vi "Autonomous Independent (1).vi"() -> ()   [LabVIEW 2016]
doc: "This VI is called when autonomous begins, and will automatically be terminated when autonomous ends. You can carry out timed or sensor driven robot movement independently without needing to return to the caller."
uses:
  <vilib>/Rock Robotics/WPI/Utilities/WPI_GetSetVariantRefNum.vi
  <vilib>/Rock Robotics/Network Tables/NT Read String.vi
  <vilib>/Rock Robotics/Network Tables/NT Write Numeric Array.vi
  <vilib>/Rock Robotics/WPI/RobotDrive/WPI_RobotDriveArcadeDrive_Standard(NoSaturation).vi
  Robot Global Data.vi
  <vilib>/Rock Robotics/Network Tables/NT Write Number.vi
  <vilib>/Rock Robotics/WPI/Counter/WPI_CounterDigitalInputToDigitalSource.vi
  <vilib>/Rock Robotics/SystemInterfaces/DIO/FPGA_DIOChannel.ctl
panel:
  out "Hook found 2":bool
  out "Degrees to turn 2":dbl
  out "Pixels to turn 2":dbl
  out "Hook Center 2":dbl
  out "Initial Hook Center 3":dbl
  out "Initial Hook Found 2":bool
  out "Distance to wall (in) 2":dbl
  out "Hook Center Cons":dbl
  out "Initial Hook Center 2":dbl
  out "Hook Center":dbl
  out "Initial Hook Found":bool
  out "Pixels to turn":dbl
  out "Move forward? S 5":bool
  out "Move forward? S4":bool
  out "Move forward? S 3":bool
  out "Move forward? S2":bool
  out "Move forward? S1":bool
  out "Distance to wall (in)":dbl
  out "Degrees to turn":dbl
  out "Hook found":bool
  out "gyro":dbl
  out "sonar distance (inches)":dbl
  out "Hook Found In False Case 2":bool
  out "gyro step  four":dbl
  out "gyro step  three":dbl
  out "gyro step two":dbl
  out "gyro step one":dbl
  out "Step 3":bool
  out "Step 2":bool
  out "Step 1":bool
  out "Encoder Loop":dbl
  out "Encoder Loop":string
  out "S2 Encoder":dbl
  out "Encoder Direction 2":string
  out "S1 Encoder inches":dbl
  out "Encoder Direction":string
  out "Current Movement, for debugging 2":T1 {"Y Joystick Value" scale=1.0..-1.0; "X Joystick Value" scale=-1.0..1.0}
  in  "Array of robot movements 2":T2(array[cluster])=[{"X Joystick Value"=0.39393939393939403, "Y Joystick Value"=0.0, "Delay (sec)"=1.0, "Movement Name"="turn"}, {"X Joystick Value"=-0.3737373737373737, "Y Joystick Value"=0.0, "Delay (sec)"=1.0, "Movement Name"="turn back"}] {"Y Joystick Value" scale=1.0..-1.0; "X Joystick Value" scale=-1.0..1.0}
  out "Motor Values":dbl[](array[numeric])
  out "Switch Pressed":bool
  out "Current Movement, for debugging":T1 {"Y Joystick Value" scale=1.0..-1.0; "X Joystick Value" scale=-1.0..1.0}
  in  "Array of robot movements":T2(array[cluster])=[{"X Joystick Value"=0.39393939393939403, "Y Joystick Value"=0.0, "Delay (sec)"=1.0, "Movement Name"="turn"}, {"X Joystick Value"=-0.3737373737373737, "Y Joystick Value"=0.0, "Delay (sec)"=1.0, "Movement Name"="turn back"}] {"Y Joystick Value" scale=1.0..-1.0; "X Joystick Value" scale=-1.0..1.0}
  # "Sensor Readings\nConstanly updated in\nwhile loopes"
  # "Be sure to right-click and choose Data Operations>>Make Current Value default if you want to save the array values with the VI"
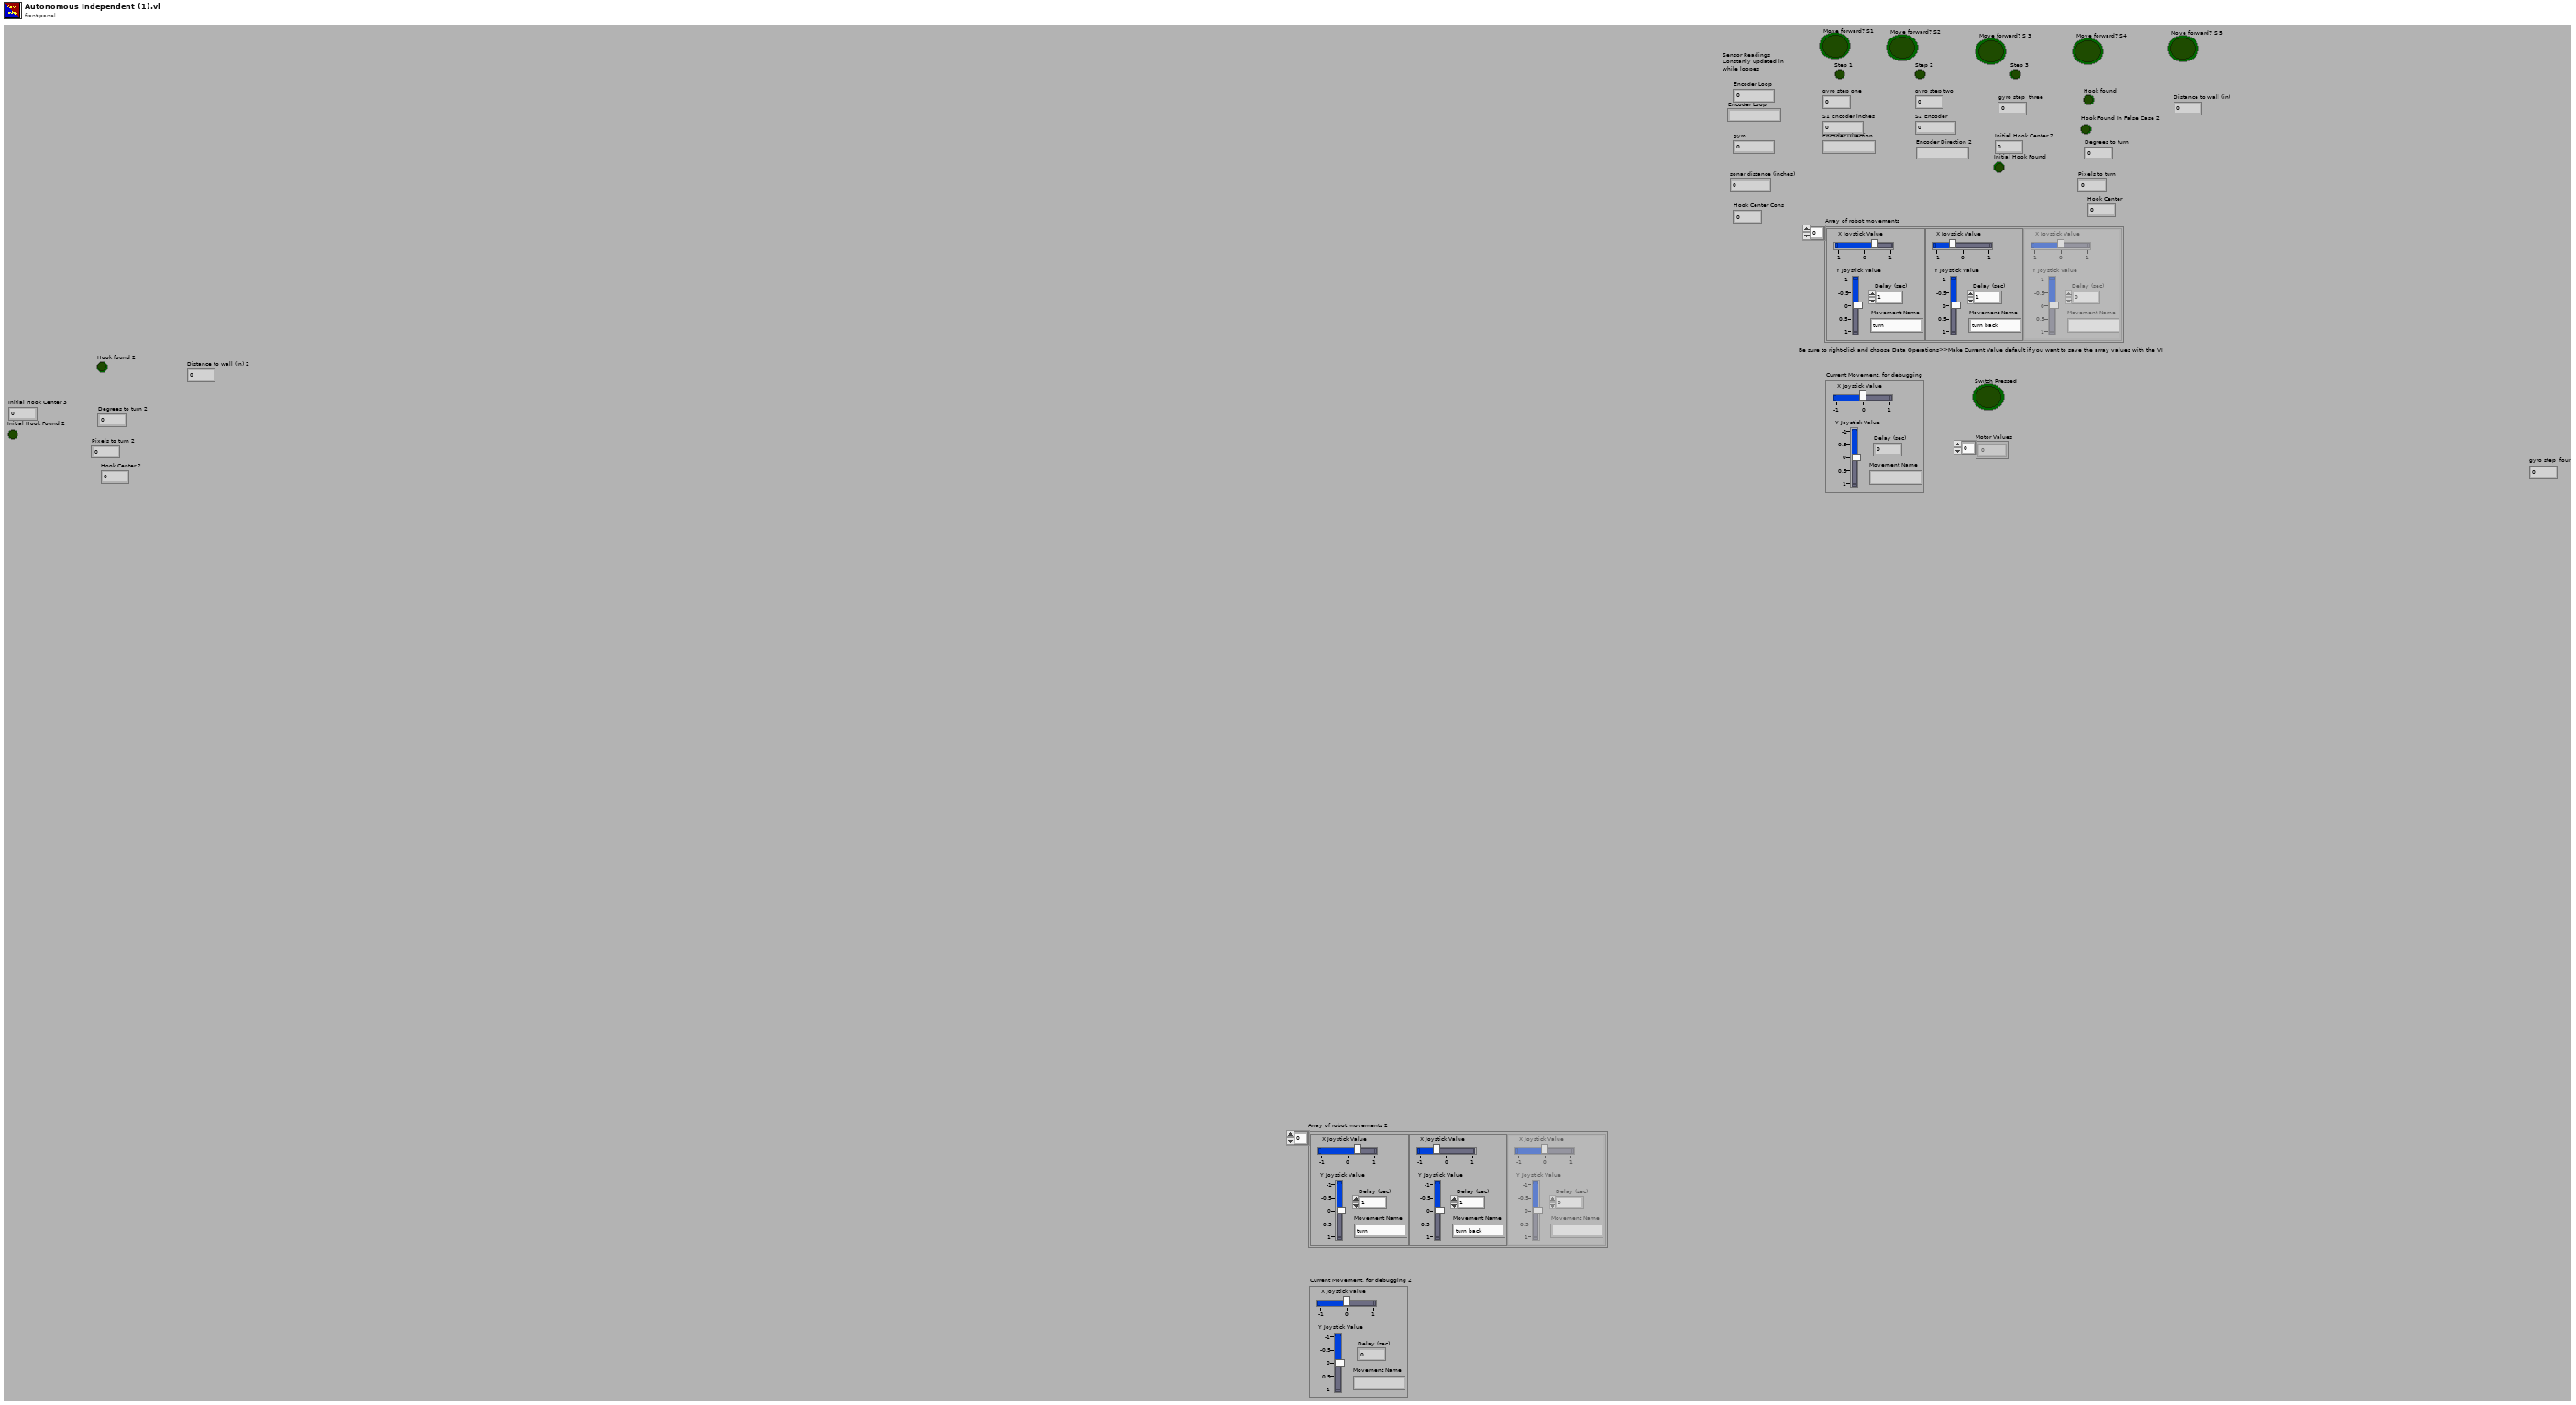
[diagram p1: front panel]
types:
  T1 = cluster{"X Joystick Value":dbl, "Y Joystick Value":dbl, "Delay (sec)":dbl, "Movement Name":string}
  T2 = cluster{"X Joystick Value":dbl, "Y Joystick Value":dbl, "Delay (sec)":dbl, "Movement Name":string}[]
  T3 = typedef "FPGA_DIOChannel.ctl" = enum8{"DIO 0", "DIO 1", "DIO 2", "DIO 3", "DIO 4", "DIO 5", "DIO 6", "DIO 7", "DIO 8", "DIO 9", "DIO MXP 0", "DIO MXP 1", "DIO MXP 2", "DIO MXP 3", "DIO MXP 4", "DIO MXP 5", "DIO MXP 6", "DIO MXP 7", "DIO MXP 8", "DIO MXP 9", "DIO MXP 10", "DIO MXP 11", "DIO MXP 12", "DIO MXP 13", "DIO MXP 14", "DIO MXP 15", "SPI Port CS1", "SPI Port CS2", "SPI Port CS3", "SPI Port MISO", "SPI Port MOSI", "Invalid"}
  T4 = typedef "WPI_DigitalInputDevRef.ctl" = cluster{"DevStatus":errorcluster, "DIO Channel":T3}
  T5 = typedef "FPGA_CounterEncoderSourceConvertionLVSourceType.ctl" = cluster{"DevStatus":errorcluster, "AnalogTriggerMode?":bool, "DigitalMode":cluster{"DIO Channel":T6}, "AnalogTriggerMode":cluster{"AnalogTriggerIndex":T7, "OutputType":T8}}
  T6 = typedef "FPGA_DIODigitalSourceChannel.ctl" = enum8{"DIO 0", "DIO 1", "DIO 2", "DIO 3", "DIO 4", "DIO 5", "DIO 6", "DIO 7", "DIO 8", "DIO 9", "DIO MXP 0", "DIO MXP 1", "DIO MXP 2", "DIO MXP 3", "DIO MXP 4", "DIO MXP 5", "DIO MXP 6", "DIO MXP 7", "DIO MXP 8", "DIO MXP 9", "DIO MXP 10", "DIO MXP 11", "DIO MXP 12", "DIO MXP 13", "DIO MXP 14", "DIO MXP 15", "Disabled"}
  T7 = typedef "FPGA_AnalogTriggerIndex.ctl" = enum8{"Trig 0", "Trig 1", "Trig 2", "Trig 3", "Trig 4", "Trig 5", "Trig 6", "Trig 7", "Invalid"}
  T8 = typedef "FPGA_AnalogTriggerOutType.ctl" = enum16{"InWindow", "TriggerState", "Rising", "Falling"}
  T9 = typedef "WPI_EncoderDevRef.ctl" = cluster{"DevStatus":errorcluster, "EncoderIndex":T10, "CounterIndex":T11, "DistancePerCount":dbl, "Decoding Type":T12}
  T10 = typedef "FPGA_EncoderIdx.ctl" = enum8{"Enc 0", "Enc 1", "Enc 2", "Enc 3", "Enc 4", "Enc 5", "Enc 6", "Enc 7", "Invalid"}
  T11 = typedef "FPGA_CounterCtrSystemIndex.ctl" = enum8{"Ctr 0", "Ctr 1", "Ctr 2", "Ctr 3", "Ctr 4", "Ctr 5", "Ctr 6", "Ctr 7", "Invalid"}
  T12 = typedef "WPI_EncoderType.ctl" = enum16{"1x", "2x", "4x"}
  T13 = typedef "WPI_JoystickDevRef.ctl" = cluster{"Device":T14}
  T14 = typedef "WPI_JoystickDeviceEnum.ctl" = enum16{"USB 0", "USB 1", "USB 2", "USB 3", "USB 4", "USB 5"}
  T15 = typedef "WPI_DriverStationPositionInfo.ctl" = enum16{"1", "2", "3"}
  T16 = typedef "WPI_RobotDriveDevRef.ctl" = cluster{"DevStatus":errorcluster, "Motors[]":T17[], "Square Inputs":bool, "Max Output":dbl}
  T17 = typedef "WPI_MotorControlDeviceRef.ctl" = cluster{"DeviceStatus":errorcluster, "Type":T18, "PWM":cluster{"PWM Channel":T19, "DeadBand":T20}, "CAN":cluster{"Device Number":u8, "SetOutput VI Ref":variant, "GetOutput VI Ref":variant, "Enable VI Ref":variant, "Disable VI Ref":variant, "Data":variant}, "Invert":bool}
  T18 = typedef "WPI_MotorControlType.ctl" = enum16{"PWM", "CAN"}
  T19 = typedef "FPGA_DIOPWMChannel.ctl" = enum8{"PWM 0", "PWM 1", "PWM 2", "PWM 3", "PWM 4", "PWM 5", "PWM 6", "PWM 7", "PWM 8", "PWM 9", "PWM MXP 0", "PWM MXP 1", "PWM MXP 2", "PWM MXP 3", "PWM MXP 4", "PWM MXP 5", "PWM MXP 6", "PWM MXP 7", "PWM MXP 8", "PWM MXP 9", "Invalid"}
  T20 = typedef "WPI_PWMDeadband.ctl" = cluster{"Name":string, "maxPositivePwm":i32, "minPositivePwm":i32, "centerPwm":i32, "maxNegativePwm":i32, "minNegativePwm":i32, "angularRange":u16}
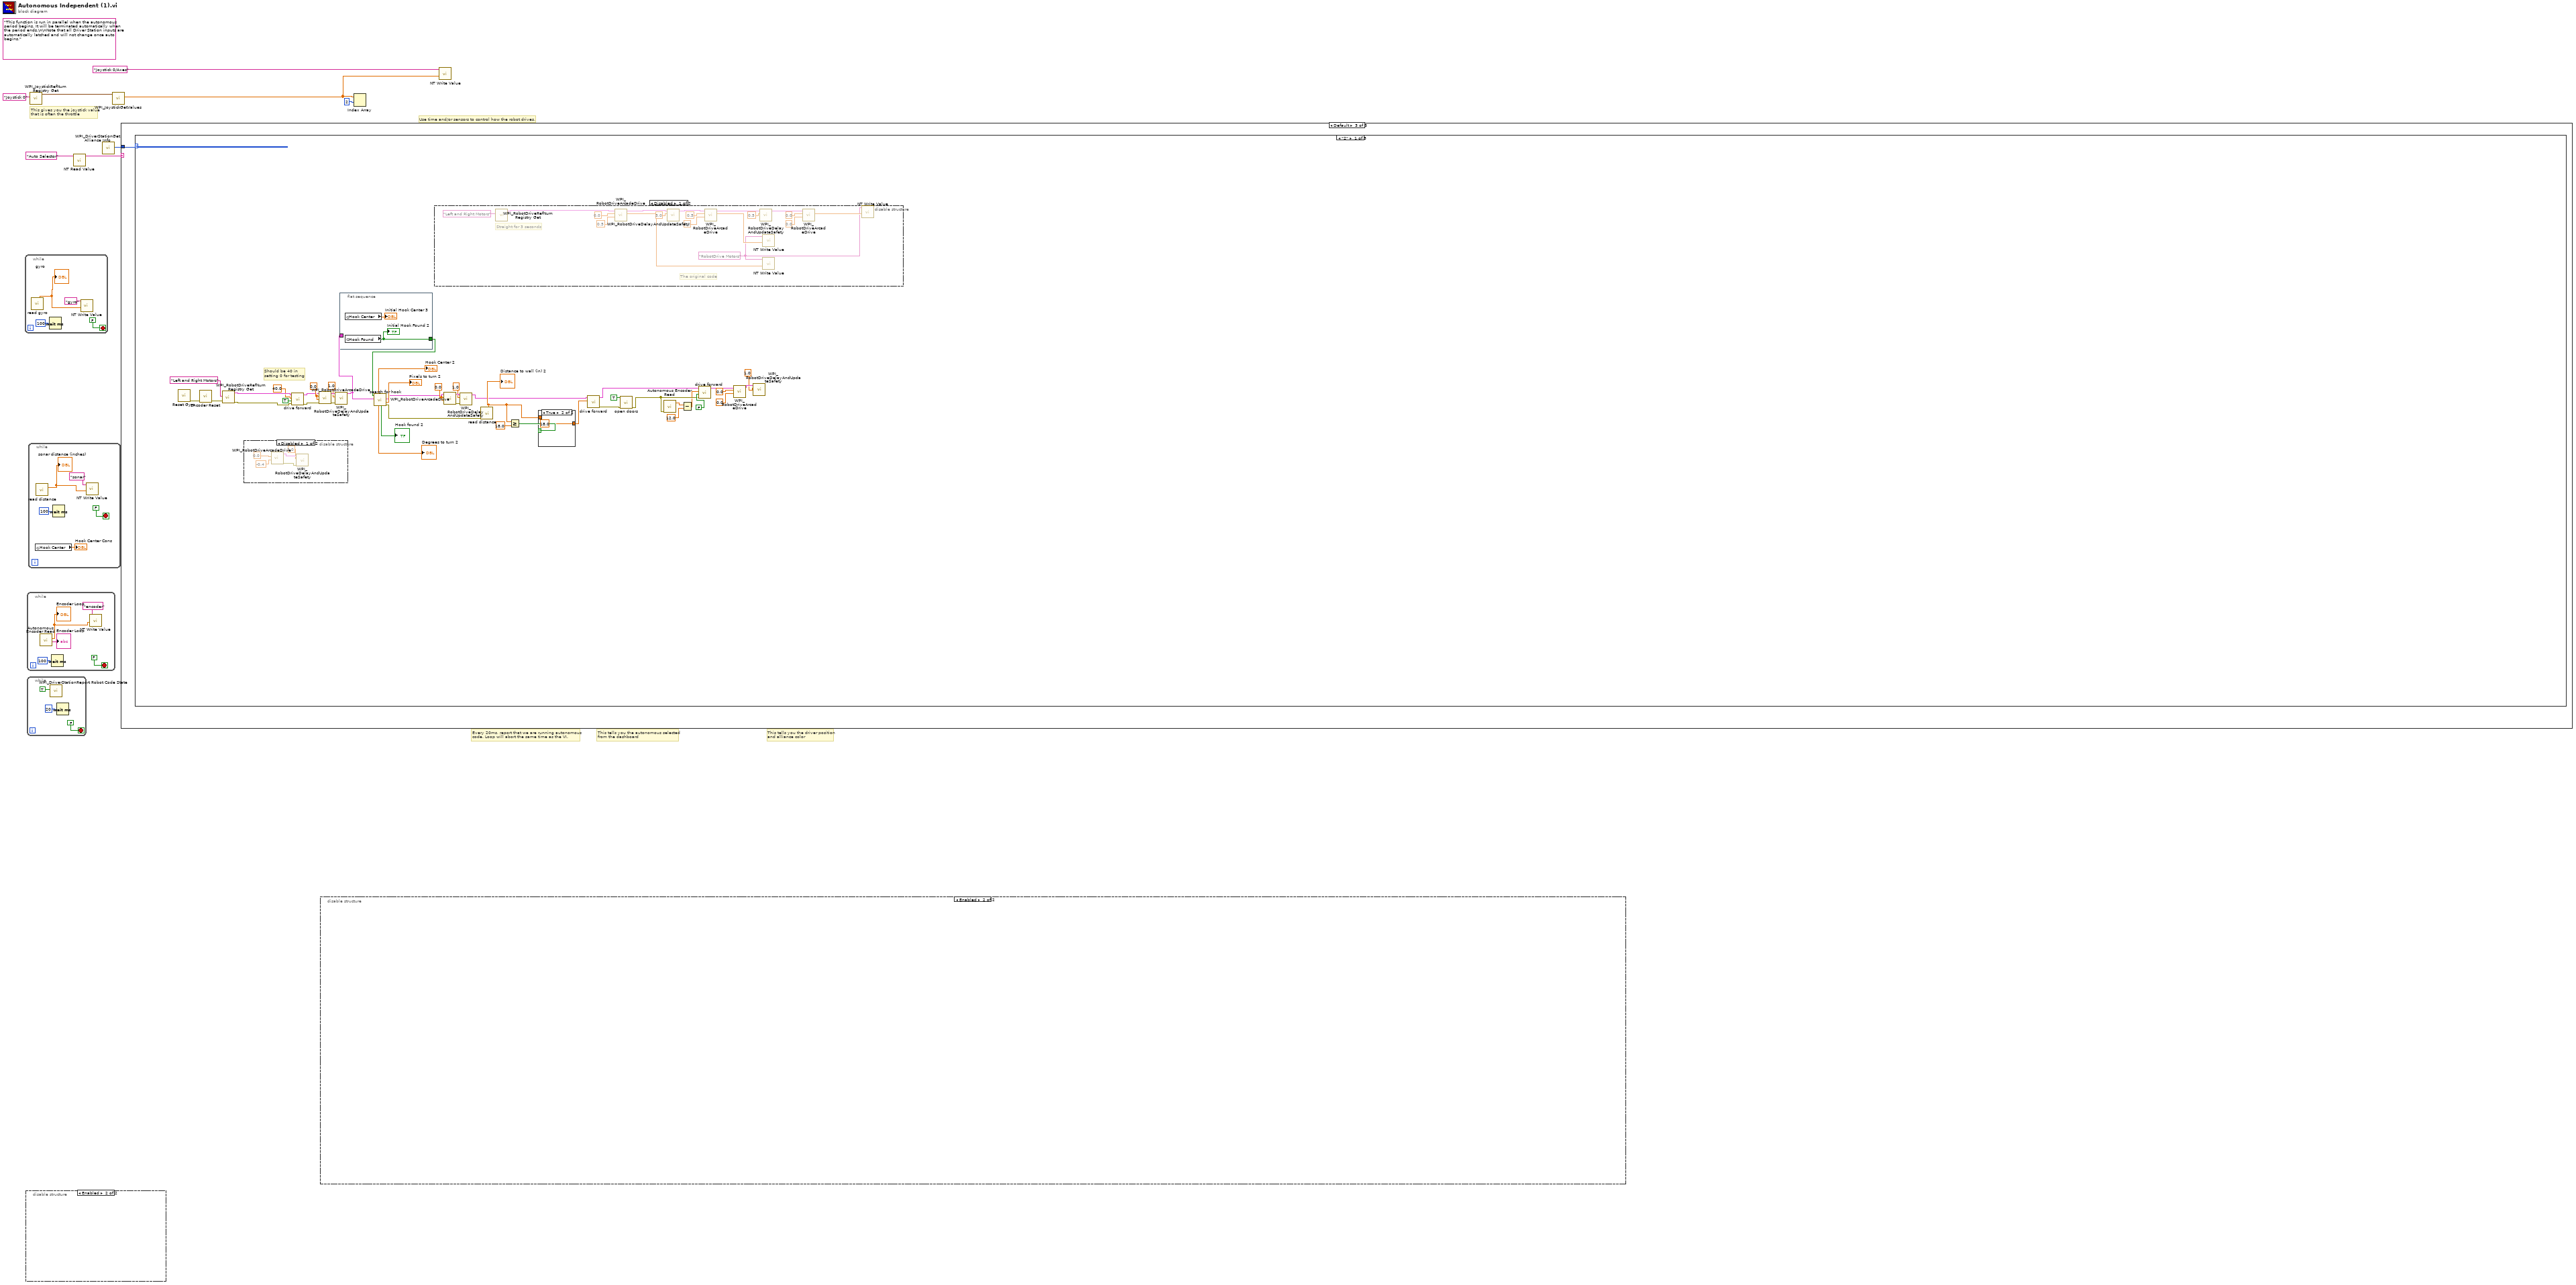
[diagram p0: block diagram]
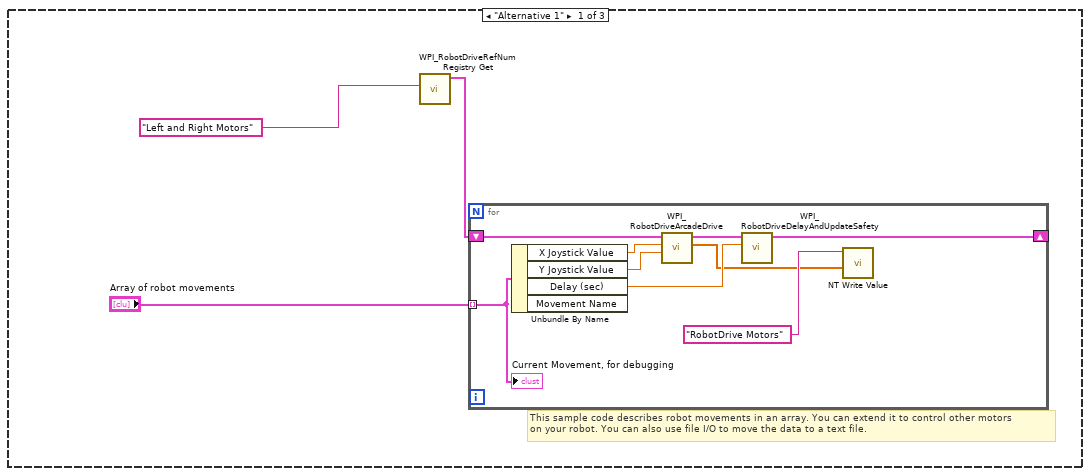
[diagram p2: hidden frame]
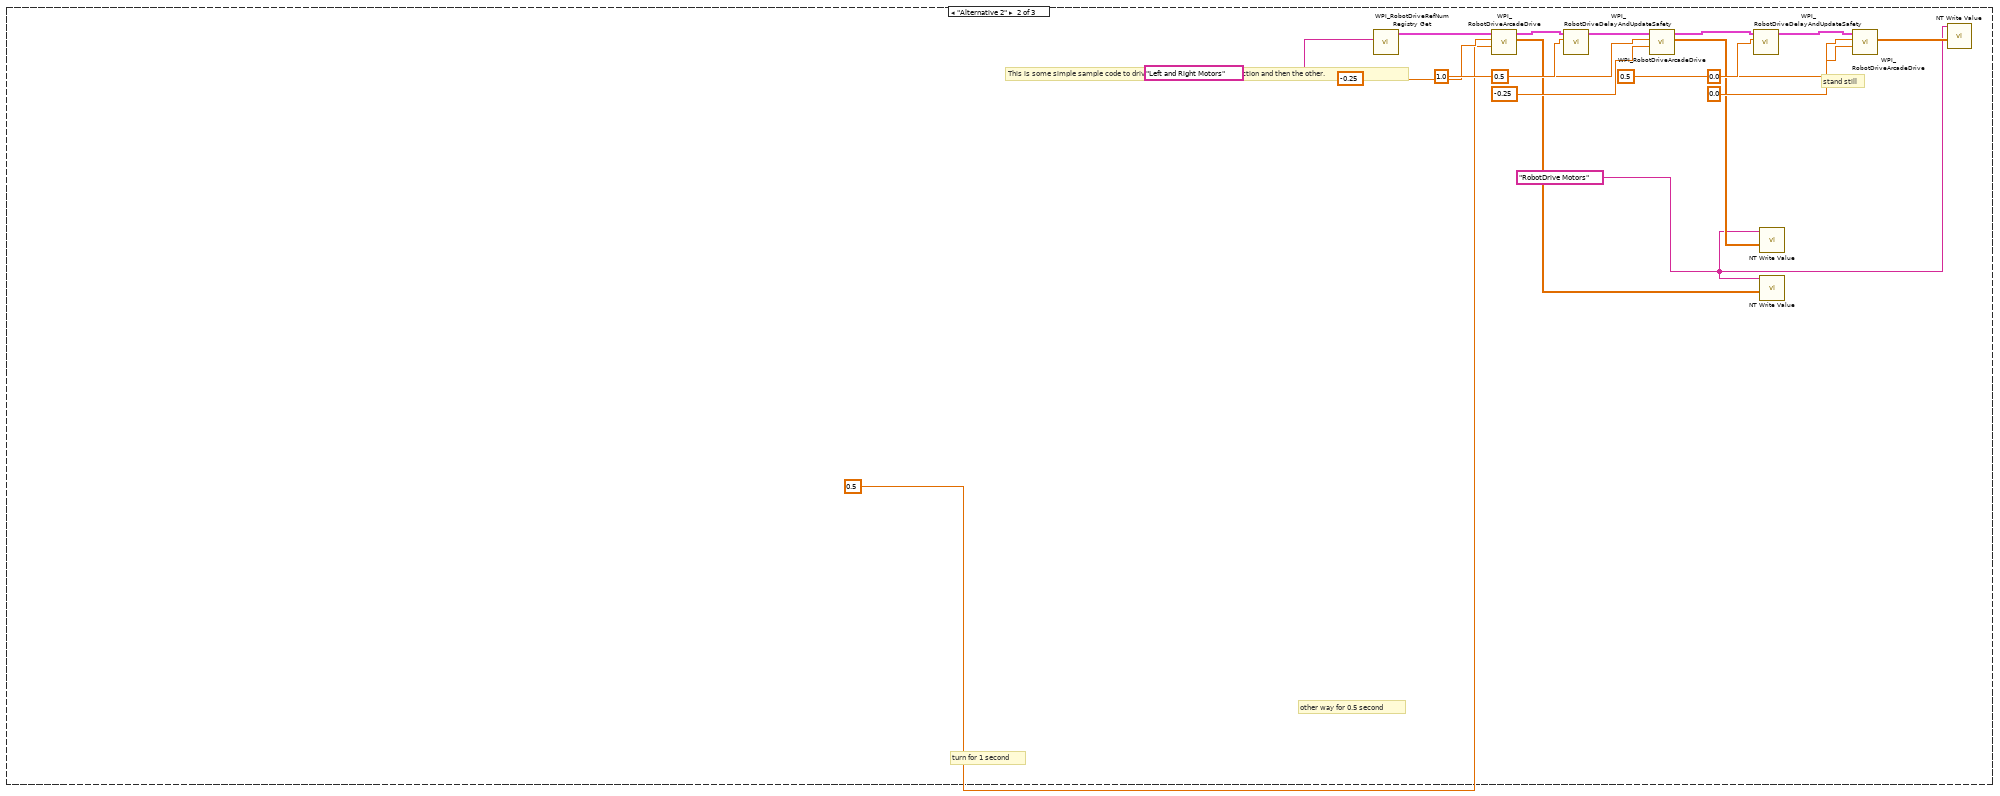
[diagram p3: hidden frame]
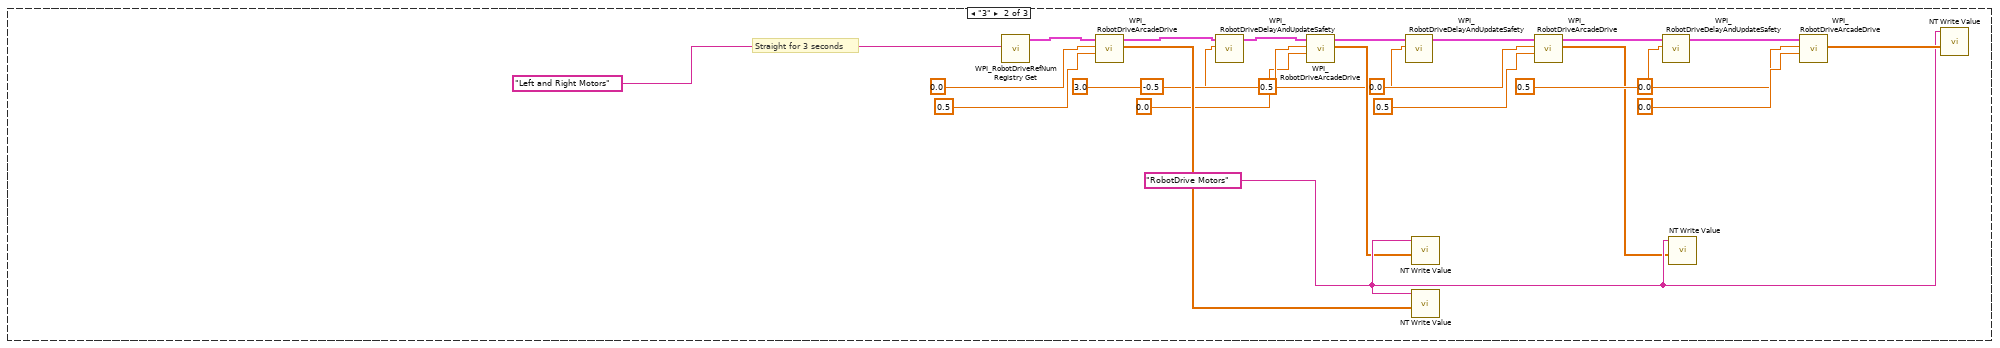
[diagram p7: hidden frame]
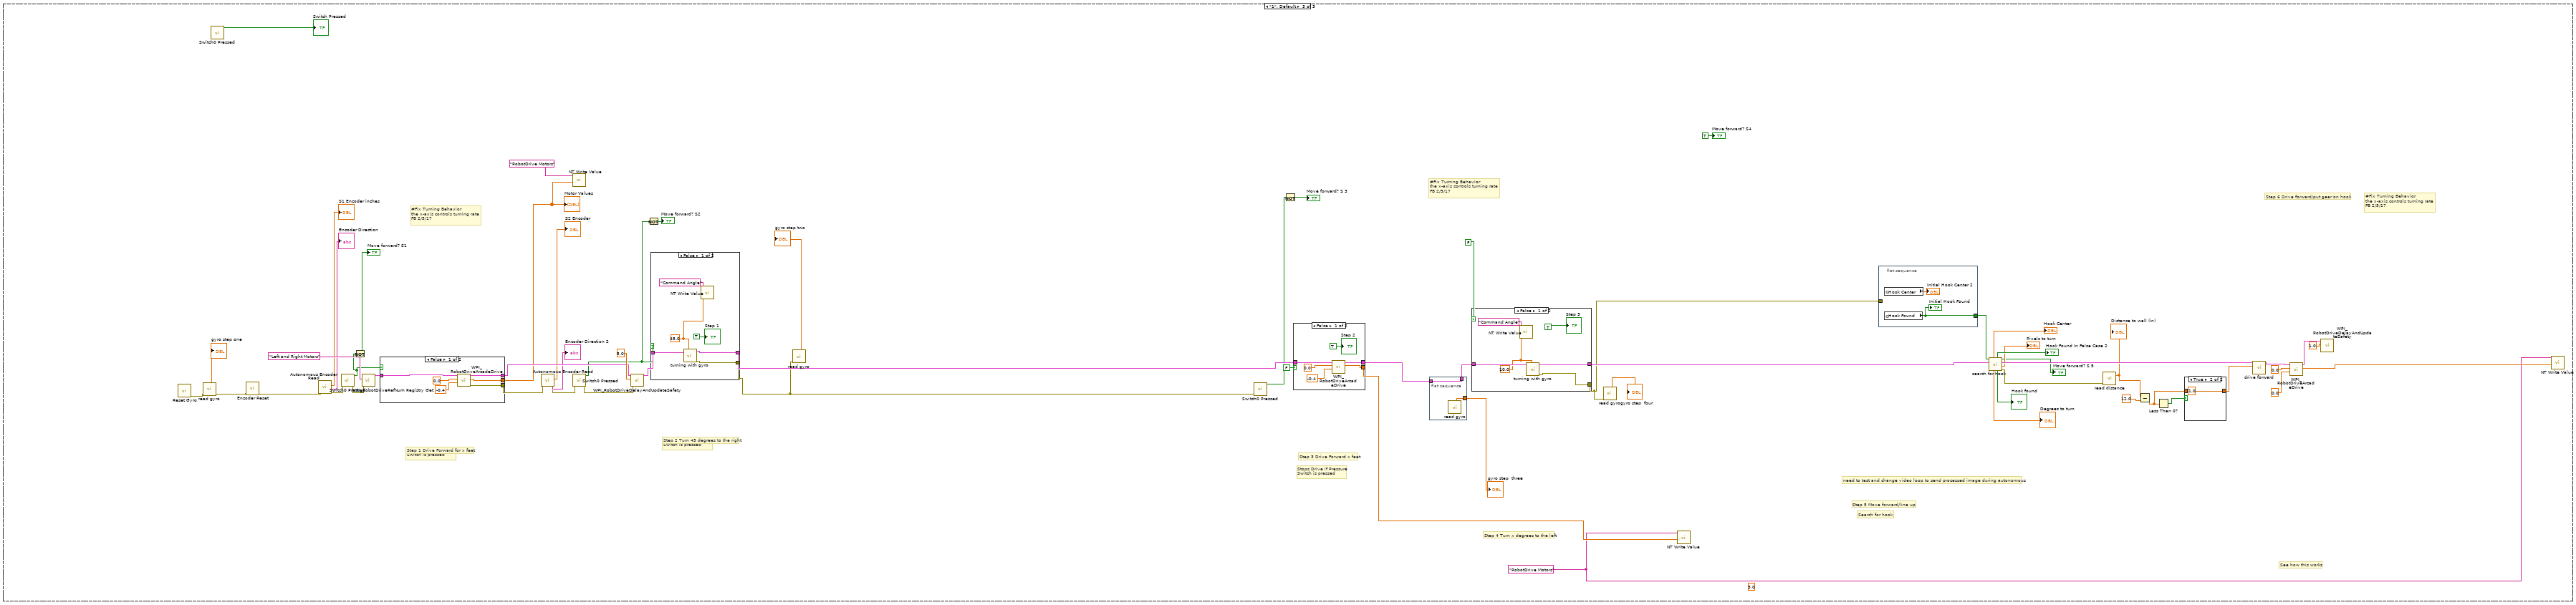
[diagram p8: hidden frame]
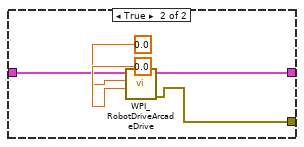
[diagram p10: hidden frame]
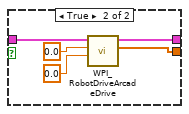
[diagram p11: hidden frame]
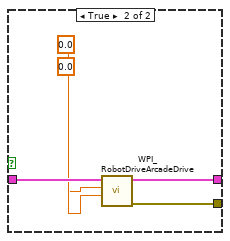
[diagram p12: hidden frame]
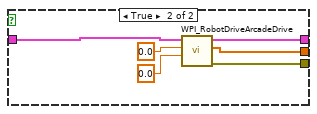
[diagram p13: hidden frame]
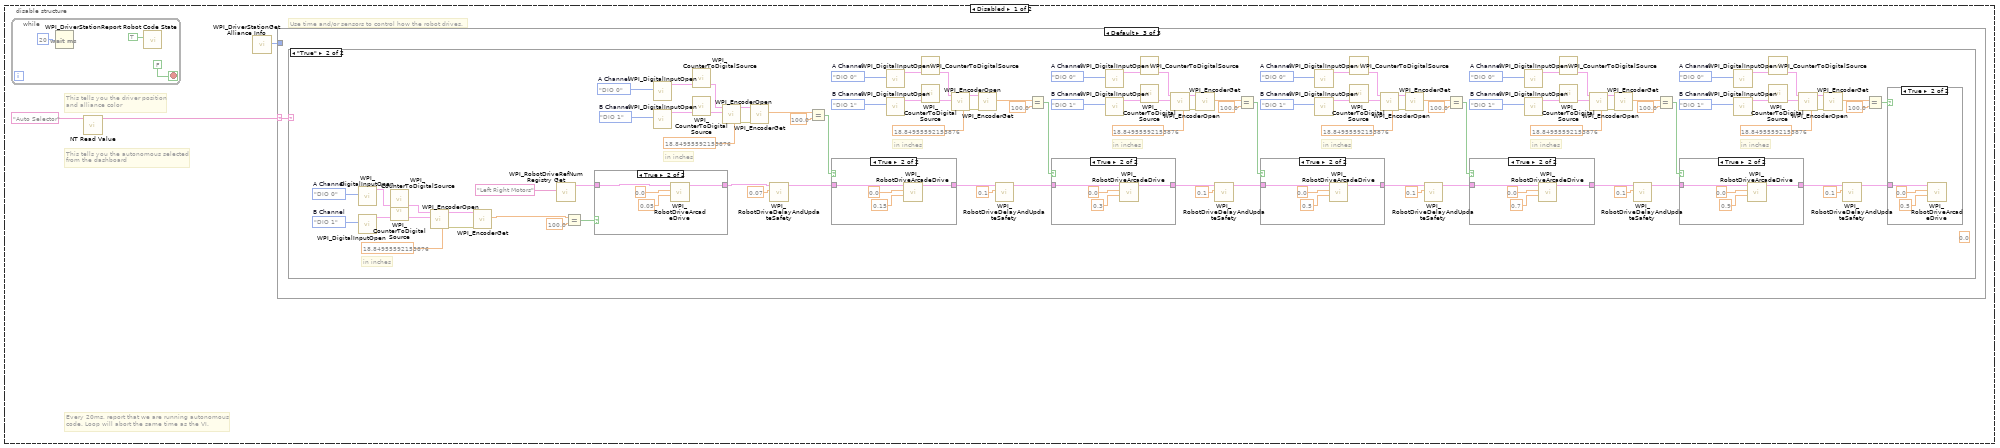
[diagram p14: hidden frame]
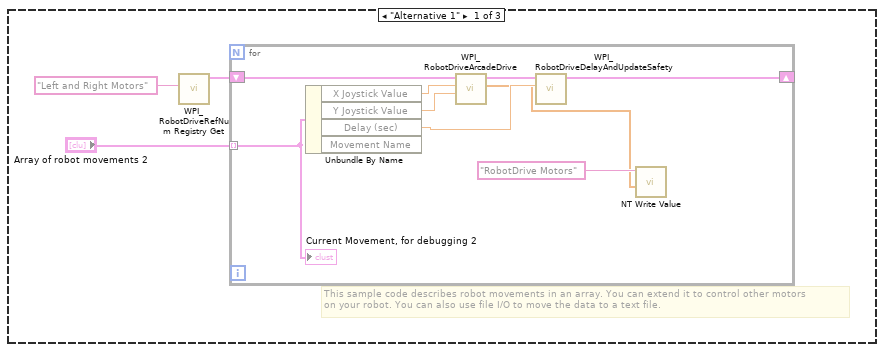
[diagram p15: hidden frame]
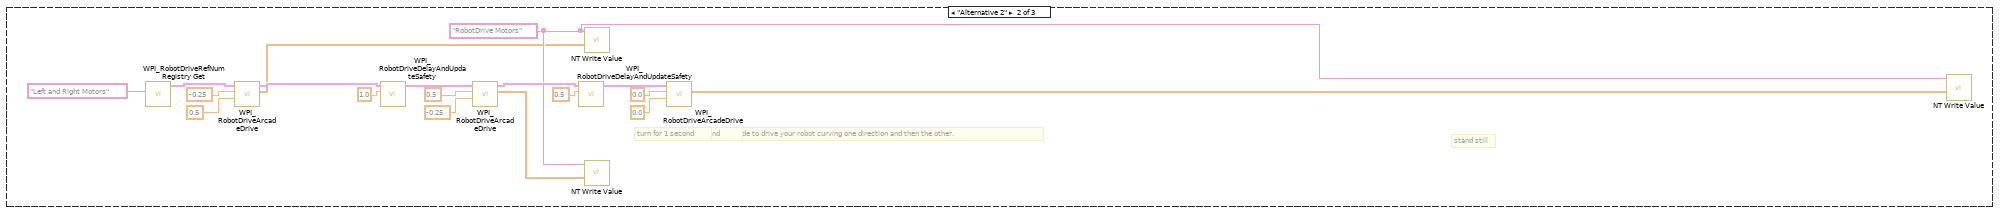
[diagram p16: hidden frame]
diagram:
  (unwired) "This function is run in parallel when the autonomous period begins. It will be terminated automatically when the period ends.\n\nNote that all Driver Station inputs are automatically latched and will not change once auto begins."
  # "This tells you the autonomous selected\nfrom the dashboard"
  # "Every 20ms, report that we are running autonomous\ncode. Loop will abort the same time as the VI."
  # "This gives you the joystick value\nthat is often the throttle"
  # "Use time and/or sensors to control how the robot drives."
  # "This tells you the driver position\nand alliance color"
  n1 = while {
    stop <- FALSE stop-if-true
    n2 = call "read gyro.vi"() -> ("Angle 2"=w10:dbl)  [unwired: 10 in, 1 out]
    "gyro" <- w10
    n3 = Wait (ms)(milliseconds to wait=u32 100) -> ()  [unwired: 1 out]
    n4 = call-poly <vilib>:"NT Write Value.vi"("Numeric"=w10, "Name"="gyro") -> ()  [unwired: 9 in, 1 out]
  }
  n5 = disable-structure shown="Enabled" {
    frame Disabled {
      w26 = FPGA_DIOChannel."DIO 1"  # B Channel
      w25 = FPGA_DIOChannel."DIO 0"  # A Channel
      # "in inches"
      n6 = call <vilib>:"WPI_DigitalInputOpen.vi"("DIO Channel"=w25) -> ("DigitalInputDevRef"=w22:T4)  [unwired: 1 in, 9 out]
      n7 = call <vilib>:"WPI_DigitalInputOpen.vi"("DIO Channel"=w26) -> ("DigitalInputDevRef"=w23:T4)  [unwired: 1 in, 9 out]
      n8 = call-poly <vilib>:"WPI_CounterToDigitalSource.vi"("DigitalInputDevRef"=w22) -> ("Digital Source"=w21:T5)  [unwired: 6 out]
      n9 = call-poly <vilib>:"WPI_CounterToDigitalSource.vi"("DigitalInputDevRef"=w23) -> ("Digital Source"=w24:T5)  [unwired: 6 out]
      n10 = call <vilib>:"WPI_EncoderOpen.vi"("DistancePerCount"=18.84955592153876, "Invert Direction (False)"=FALSE, "BSource"=w24, "ASource"=w21) -> ("error out"=w19:errorcluster, "EncoderDevRef"=w20:T9)  [unwired: 4 in, 2 out]
      n11 = call-poly <vilib>:"NT Write Value.vi"("Name"="Encoder Distance") -> ()  [unwired: 10 in, 1 out]
      n12 = call <vilib>:"WPI_EncoderRefNum Registry Set.vi"("error in (no error)"=w19, "refnum name"="Encoder", "EncoderDevRef"=w20) -> ("error out"=w17:errorcluster, "EncoderDevRef"=w18:T9)  [unwired: 7 in]
      n13 = call <vilib>:"WPI_EncoderGet.vi"("error in (no error)"=w17, "EncoderDevRef"=w18) -> ()  [unwired: 4 in, 6 out]
    }
    frame Enabled {
    }
  }
  n14 = while {
    stop <- FALSE stop-if-true
    n15 = call "Autonomous Encoder Read.vi"() -> ("Encoder Direction"=→"Encoder Loop":string, "Encoder Distance"=w28:dbl)  [unwired: 9 in, 1 out]
    "Encoder Loop" <- w28
    n16 = Wait (ms)(milliseconds to wait=u32 100) -> ()  [unwired: 1 out]
    n17 = call-poly <vilib>:"NT Write Value.vi"("Numeric"=w28, "Name"="encoder") -> ()  [unwired: 9 in, 1 out]
  }
  n18 = while {
    stop <- FALSE stop-if-true
    n19 = call <vilib>:"WPI_DriverStationReport Robot Code State.vi"("Autonomous"=TRUE) -> ()  [unwired: 10 in, 1 out]
    n20 = Wait (ms)(milliseconds to wait=u32 20) -> ()  [unwired: 1 out]
  }
  n21 = while {
    stop <- FALSE stop-if-true
    n22 = global read "Robot Global Data.vi" "Hook Center"() -> (→"Hook Center Cons":dbl)
    n23 = call "read distance.vi"() -> ("Distance 2"=w37:dbl)  [unwired: 10 in, 1 out]
    "sonar distance (inches)" <- w37
    n24 = Wait (ms)(milliseconds to wait=u32 100) -> ()  [unwired: 1 out]
    n25 = call-poly <vilib>:"NT Write Value.vi"("Numeric"=w37, "Name"="sonar") -> ()  [unwired: 9 in, 1 out]
  }
  n26 = call <vilib>:"WPI_JoystickRefNum Registry Get.vi"("refnum name"="Joystick 0") -> ("JoystickDevRef"=w7:T13)  [unwired: 1 in, 9 out]
  n27 = call-poly <vilib>:"NT Read Value.vi"("Name"="Auto Selector") -> ("String"=w4:string)  [unwired: 9 in, 1 out]
  n28 = call <vilib>:"WPI_DriverStationGet Alliance Info.vi"() -> ("Position"=w1:T15)  [unwired: 11 out]
  n29 = call <vilib>:"WPI_JoystickGetValues.vi"("JoystickDevRef"=w7) -> ("Axes"=w3:dbl[])  [unwired: 6 in, 4 out]
  n30 = case shown="Default" w4 {
    tunnel: w1 -> [_ _ w70]
    frame "Alternative 1" {
      # "This sample code describes robot movements in an array. You can extend it to control other motors\non your robot. You can also use file I/O to move the data to a text file."
      n31 = call <vilib>:"WPI_RobotDriveRefNum Registry Get.vi"("refnum name"="Left and Right Motors") -> ("RobotDriveDevRef"=w41:T16)  [unwired: 1 in, 9 out]
      n32 = for {
        shift-right: [w49] -> _
        shift-left: w41 -> [w50]
        tunnel: "Array of robot movements" -> [w45] mode=indexing
        n33 = Unbundle By Name(w45) -> ("X Joystick Value"=w48:dbl, "Y Joystick Value"=w47:dbl, "Delay (sec)"=w46:dbl)  [unwired: 1 out]
        n34 = call-poly <vilib>:"WPI_RobotDriveArcadeDrive.vi"("Y axis value"=w47, "X axis value"=w48, "RobotDriveDevRef"=w50) -> ("Motor Values"=w43:dbl[], "RobotDriveDevRef"=w51:T16)  [unwired: 1 in, 6 out]
        n35 = call <vilib>:"WPI_RobotDriveDelayAndUpdateSafety.vi"("Delay (s)"=w46, "RobotDriveDevRef"=w51) -> ("RobotDriveDevRef 2"=w49:T16)  [unwired: 8 in, 1 out]
        n36 = call-poly <vilib>:"NT Write Value.vi"("Numeric Array"=w43, "Name"="RobotDrive Motors") -> ()  [unwired: 9 in, 1 out]
        "Current Movement, for debugging" <- w45
      }
    }
    frame "Alternative 2" {
      w53 = "RobotDrive Motors" ("Name")
      # "This is some simple sample code to drive your robot curving one direction and then the other."
      # "stand still"
      # "other way for 0.5 second"
      # "turn for 1 second"
      n37 = call <vilib>:"WPI_RobotDriveRefNum Registry Get.vi"("refnum name"="Left and Right Motors") -> ("RobotDriveDevRef"=w69:T16)  [unwired: 1 in, 9 out]
      n38 = call-poly <vilib>:"WPI_RobotDriveArcadeDrive.vi"("Y axis value"=0.5 ("X axis value"), "X axis value"=-0.25, "RobotDriveDevRef"=w69) -> ("Motor Values"=w52:dbl[], "RobotDriveDevRef"=w62:T16)  [unwired: 1 in, 6 out]
      n39 = call <vilib>:"WPI_RobotDriveDelayAndUpdateSafety.vi"("Delay (s)"=1.0, "RobotDriveDevRef"=w62) -> ("RobotDriveDevRef 2"=w63:T16)  [unwired: 8 in, 1 out]
      n40 = call-poly <vilib>:"WPI_RobotDriveArcadeDrive.vi"("Y axis value"=-0.25 ("X axis value"), "X axis value"=0.5, "RobotDriveDevRef"=w63) -> ("Motor Values"=w54:dbl[], "RobotDriveDevRef"=w64:T16)  [unwired: 1 in, 6 out]
      n41 = call <vilib>:"WPI_RobotDriveDelayAndUpdateSafety.vi"("Delay (s)"=0.5, "RobotDriveDevRef"=w64) -> ("RobotDriveDevRef 2"=w65:T16)  [unwired: 8 in, 1 out]
      n42 = call-poly <vilib>:"NT Write Value.vi"("Numeric Array"=w54, "Name"=w53) -> ()  [unwired: 9 in, 1 out]
      n43 = call-poly <vilib>:"NT Write Value.vi"("Numeric Array"=w52, "Name"=w53) -> ()  [unwired: 9 in, 1 out]
      n44 = call-poly <vilib>:"WPI_RobotDriveArcadeDrive.vi"("Y axis value"=0.0 ("X axis value"), "X axis value"=0.0, "RobotDriveDevRef"=w65) -> ("Motor Values"=w55:dbl[])  [unwired: 1 in, 7 out]
      n45 = call-poly <vilib>:"NT Write Value.vi"("Numeric Array"=w55, "Name"=w53) -> ()  [unwired: 9 in, 1 out]
    }
    frame Default {
      n46 = case shown="\"2\"" w70 {
        frame "2" {
          w73 = 0.0 ("X axis value")
          w80 = 0.0 ("X axis value")
          # "Should be 40 in\nsetting 0 for testing"
          n47 = call "Reset Gyro.vi"() -> ("error out"=w92:errorcluster)  [unwired: 11 in]
          n48 = call "Encoder Reset.vi"("error in (no error)"=w92) -> ("error out"=w103:errorcluster)  [unwired: 10 in]
          n49 = call <vilib>:"WPI_RobotDriveRefNum Registry Get.vi"("error in (no error)"=w103, "refnum name"="Left and Right Motors") -> ("error out"=w91:errorcluster, "RobotDriveDevRef"=w102:T16)  [unwired: 8 out]
          n50 = disable-structure shown="Disabled" {
            frame Disabled {
              n51 = call-poly <vilib>:"WPI_RobotDriveArcadeDrive.vi"("Y axis value"=-0.4 ("X axis value"), "X axis value"=0.0) -> ("error out"=w115:errorcluster, 3:"RobotDriveDevRef"=w116:T16, 11:"RobotDriveDevRef"=w117:T16)  [unwired: 1 in, 6 out]
              n52 = call <vilib>:"WPI_RobotDriveDelayAndUpdateSafety.vi"("error in (no error)"=w115, "Delay (s)"=3.0, "RobotDriveDevRef"=w116) -> ()  [unwired: 7 in, 2 out]
            }
            frame Enabled {
            }
          }
          n53 = call "drive forward.vi"("error in (no error)"=w91, "forward"=TRUE, "desired distance"=40.0, "RobotDriveDevRef in"=w102) -> ("error out"=w78:errorcluster, "RobotDriveDevRef out"=w79:T16)  [unwired: 6 in]
          n54 = call-poly <vilib>:"WPI_RobotDriveArcadeDrive.vi"("error in (no error)"=w78, "Y axis value"=w80, "X axis value"=w80, "RobotDriveDevRef"=w79) -> ("error out"=w82:errorcluster, "RobotDriveDevRef"=w83:T16)  [unwired: 6 out]
          n55 = call <vilib>:"WPI_RobotDriveDelayAndUpdateSafety.vi"("error in (no error)"=w82, "Delay (s)"=1.0, "RobotDriveDevRef"=w83) -> ("RobotDriveDevRef 2"=w77:T16)  [unwired: 7 in, 1 out]
          n56 = flat-sequence {
            tunnel: [w120] -> w109
            tunnel: w77 -> [_]
            frame #0 {
              n57 = global read "Robot Global Data.vi" "Hook Center"() -> (→"Initial Hook Center 3":dbl)
              n58 = global read "Robot Global Data.vi" "Hook Found"() -> (w120:bool)
              "Initial Hook Found 2" <- w120
            }
          }
          n59 = call "search for hook.vi"("RobotDriveDevRef in"=w77, "Hook Found"=w109) -> ("error out"=w111:errorcluster, "Pixels to turn"=→"Pixels to turn 2":dbl, "RobotDriveDevRef out"=w71:T16, "Hook found"=→"Hook found 2":bool, "Degrees to turn"=→"Degrees to turn 2":dbl, "Hook Center"=→"Hook Center 2":dbl)  [unwired: 2 in, 2 out]
          n60 = disable-structure shown="Disabled" {
            frame Disabled {
              w125 = "RobotDrive Motors" ("Name")
              # "The original code"
              # "Straight for 3 seconds"
              n61 = call <vilib>:"WPI_RobotDriveRefNum Registry Get.vi"("refnum name"="Left and Right Motors") -> ("RobotDriveDevRef"=w141:T16)  [unwired: 1 in, 9 out]
              n62 = call-poly <vilib>:"WPI_RobotDriveArcadeDrive.vi"("Y axis value"=0.5 ("X axis value"), "X axis value"=0.0, "RobotDriveDevRef"=w141) -> ("Motor Values"=w129:dbl[], "RobotDriveDevRef"=w135:T16)  [unwired: 1 in, 6 out]
              n63 = call <vilib>:"WPI_RobotDriveDelayAndUpdateSafety.vi"("Delay (s)"=3.0, "RobotDriveDevRef"=w135) -> ("RobotDriveDevRef 2"=w136:T16)  [unwired: 8 in, 1 out]
              n64 = call-poly <vilib>:"WPI_RobotDriveArcadeDrive.vi"("Y axis value"=0.0 ("X axis value"), "X axis value"=0.5, "RobotDriveDevRef"=w136) -> ("Motor Values"=w130:dbl[], "RobotDriveDevRef"=w137:T16)  [unwired: 1 in, 6 out]
              n65 = call <vilib>:"WPI_RobotDriveDelayAndUpdateSafety.vi"("Delay (s)"=0.5, "RobotDriveDevRef"=w137) -> ("RobotDriveDevRef 2"=w124:T16)  [unwired: 8 in, 1 out]
              n66 = call-poly <vilib>:"NT Write Value.vi"("Numeric Array"=w130, "Name"=w125) -> ()  [unwired: 9 in, 1 out]
              n67 = call-poly <vilib>:"NT Write Value.vi"("Numeric Array"=w129, "Name"=w125) -> ()  [unwired: 9 in, 1 out]
              n68 = call-poly <vilib>:"WPI_RobotDriveArcadeDrive.vi"("Y axis value"=0.0 ("X axis value"), "X axis value"=0.0, "RobotDriveDevRef"=w124) -> ("Motor Values"=w126:dbl[])  [unwired: 1 in, 7 out]
              n69 = call-poly <vilib>:"NT Write Value.vi"("Numeric Array"=w126, "Name"=w125) -> ()  [unwired: 9 in, 1 out]
            }
            frame Enabled {
            }
          }
          n70 = call-poly <vilib>:"WPI_RobotDriveArcadeDrive.vi"("Y axis value"=w73, "X axis value"=w73, "RobotDriveDevRef"=w71) -> ("error out"=w75:errorcluster, "RobotDriveDevRef"=w76:T16)  [unwired: 1 in, 6 out]
          n71 = call <vilib>:"WPI_RobotDriveDelayAndUpdateSafety.vi"("error in (no error)"=w75, "Delay (s)"=1.0, "RobotDriveDevRef"=w76) -> ("RobotDriveDevRef 2"=w72:T16)  [unwired: 7 in, 1 out]
          n72 = call "read distance.vi"("error in (no error)"=w111) -> ("Distance 2"=w98:dbl)  [unwired: 9 in, 1 out]
          "Distance to wall (in) 2" <- w98
          n73 = Greater Or Equal?(x=w98, y=18.0) -> (x >= y?=w100:bool)
          n74 = case shown="True" w100 {
            tunnel: [w122 18.0 ("f")] -> w99
            tunnel: w98 -> [w122 _]
            frame False {
            }
            frame True {
            }
          }
          n75 = call "drive forward.vi"("desired distance"=w99, "RobotDriveDevRef in"=w72) -> ("error out"=w95:errorcluster, "RobotDriveDevRef out"=w94:T16)  [unwired: 8 in]
          n76 = call "open doors.vi"("error in (no error)"=w95, "Open"=TRUE) -> ("error out"=w87:errorcluster)  [unwired: 9 in]
          n77 = call "Autonomous Encoder Read.vi"("error in (no error)"=w87) -> ("Encoder Distance"=w86:dbl)  [unwired: 8 in, 2 out]
          n78 = Subtract(x=w86, y=12.0 ("desired distance")) -> (x-y=w85:dbl)
          n79 = call "drive forward.vi"("error in (no error)"=w87, "forward"=FALSE, "desired distance"=w85, "RobotDriveDevRef in"=w94) -> ("RobotDriveDevRef out"=w96:T16)  [unwired: 6 in, 1 out]
          n80 = call-poly <vilib>:"WPI_RobotDriveArcadeDrive.vi"("Y axis value"=0.0 ("X axis value"), "X axis value"=0.0, "RobotDriveDevRef"=w96) -> ("RobotDriveDevRef"=w110:T16)  [unwired: 1 in, 7 out]
          n81 = call <vilib>:"WPI_RobotDriveDelayAndUpdateSafety.vi"("Delay (s)"=1.0, "RobotDriveDevRef"=w110) -> ()  [unwired: 8 in, 2 out]
        }
        frame "3" {
          w164 = "RobotDrive Motors" ("Name")
          # "Straight for 3 seconds"
          n82 = call <vilib>:"WPI_RobotDriveRefNum Registry Get.vi"("refnum name"="Left and Right Motors") -> ("RobotDriveDevRef"=w142:T16)  [unwired: 1 in, 9 out]
          n83 = call-poly <vilib>:"WPI_RobotDriveArcadeDrive.vi"("Y axis value"=0.5 ("X axis value"), "X axis value"=0.0, "RobotDriveDevRef"=w142) -> ("Motor Values"=w158:dbl[], "RobotDriveDevRef"=w149:T16)  [unwired: 1 in, 6 out]
          n84 = call <vilib>:"WPI_RobotDriveDelayAndUpdateSafety.vi"("Delay (s)"=3.0, "RobotDriveDevRef"=w149) -> ("RobotDriveDevRef 2"=w148:T16)  [unwired: 8 in, 1 out]
          n85 = call-poly <vilib>:"WPI_RobotDriveArcadeDrive.vi"("Y axis value"=0.0 ("X axis value"), "X axis value"=-0.5, "RobotDriveDevRef"=w148) -> ("Motor Values"=w157:dbl[], "RobotDriveDevRef"=w147:T16)  [unwired: 1 in, 6 out]
          n86 = call <vilib>:"WPI_RobotDriveDelayAndUpdateSafety.vi"("Delay (s)"=0.5, "RobotDriveDevRef"=w147) -> ("RobotDriveDevRef 2"=w146:T16)  [unwired: 8 in, 1 out]
          n87 = call-poly <vilib>:"NT Write Value.vi"("Numeric Array"=w157, "Name"=w164) -> ()  [unwired: 9 in, 1 out]
          n88 = call-poly <vilib>:"NT Write Value.vi"("Numeric Array"=w158, "Name"=w164) -> ()  [unwired: 9 in, 1 out]
          n89 = call-poly <vilib>:"WPI_RobotDriveArcadeDrive.vi"("Y axis value"=0.5 ("X axis value"), "X axis value"=0.0, "RobotDriveDevRef"=w146) -> ("Motor Values"=w156:dbl[], "RobotDriveDevRef"=w162:T16)  [unwired: 1 in, 6 out]
          n90 = call <vilib>:"WPI_RobotDriveDelayAndUpdateSafety.vi"("Delay (s)"=0.5, "RobotDriveDevRef"=w162) -> ("RobotDriveDevRef 2"=w163:T16)  [unwired: 8 in, 1 out]
          n91 = call-poly <vilib>:"NT Write Value.vi"("Numeric Array"=w156, "Name"=w164) -> ()  [unwired: 9 in, 1 out]
          n92 = call-poly <vilib>:"WPI_RobotDriveArcadeDrive.vi"("Y axis value"=0.0 ("X axis value"), "X axis value"=0.0, "RobotDriveDevRef"=w163) -> ("Motor Values"=w165:dbl[])  [unwired: 1 in, 7 out]
          n93 = call-poly <vilib>:"NT Write Value.vi"("Numeric Array"=w165, "Name"=w164) -> ()  [unwired: 9 in, 1 out]
        }
        frame "1", Default {
          (unwired) 3.0 ("Delay (s)")
          w216 = "RobotDrive Motors" ("Name")
          # "See how this works"
          # "need to test and change video loop to send processed image during autonomous"
          # "#Fix Turning Behavior \nthe x-axis controls turning rate  \nFB 2/5/17"
          # "#Fix Turning Behavior \nthe x-axis controls turning rate  \nFB 2/5/17"
          # "#Fix Turning Behavior \nthe x-axis controls turning rate  \nFB 2/5/17"
          # "Search for hook"
          # "Step 6 Drive forward/put gear on hook"
          # "Step 5 Move forward/line up"
          # "Step 4 Turn x degrees to the left"
          # "Step 3 Drive Forward x feet"
          # "Step 2 Turn 45 degrees to the right"
          # "Step 1 Drive Forward for x feet"
          # "Stops Drive if Pressure\nSwitch is pressed"
          # "Stops Drive if Pressure\nSwitch is pressed"
          # "Stops Drive if Pressure\nSwitch is pressed"
          n94 = call "Reset Gyro.vi"() -> ("error out"=w175:errorcluster)  [unwired: 11 in]
          n95 = call "read gyro.vi"("error in (no error)"=w175) -> ("error out"=w174:errorcluster, "Angle 2"=→"gyro step one":dbl)  [unwired: 9 in]
          n96 = call "Switch0 Pressed.vi"() -> ("Switch Pressed"=→"Switch Pressed":bool)  [unwired: 10 in, 1 out]
          n97 = call "Encoder Reset.vi"("error in (no error)"=w174) -> ("error out"=w173:errorcluster)  [unwired: 10 in]
          n98 = call "Autonomous Encoder Read.vi"("error in (no error)"=w173) -> ("error out"=w212:errorcluster, "Encoder Direction"=→"Encoder Direction":string, "Encoder Distance"=→"S1 Encoder inches":dbl)  [unwired: 8 in]
          n99 = call "Switch0 Pressed.vi"("error in (no error)"=w212) -> ("error out"=w213:errorcluster, "Switch Pressed"=w183:bool)  [unwired: 9 in]
          n100 = Not(x=w183) -> (.not. x?=→"Move forward? S1":bool)
          n101 = call <vilib>:"WPI_RobotDriveRefNum Registry Get.vi"("error in (no error)"=w213, "refnum name"="Left and Right Motors") -> ("RobotDriveDevRef"=w226:T16)  [unwired: 9 out]
          n102 = case shown="False" w183 {
            tunnel: w226 -> [w269 w277]
            tunnel: [w270 w276] -> w222
            tunnel: [w268 w274] -> w220
            tunnel: [w266 w272] -> w205
            frame False {
              n103 = call-poly <vilib>:"WPI_RobotDriveArcadeDrive.vi"("Y axis value"=-0.4 ("X axis value"), "X axis value"=0.0, "RobotDriveDevRef"=w269) -> ("error out"=w266:errorcluster, "Motor Values"=w268:dbl[], "RobotDriveDevRef"=w270:T16)  [unwired: 1 in, 5 out]
            }
            frame True {
              n104 = call-poly <vilib>:"WPI_RobotDriveArcadeDrive.vi"("Y axis value"=0.0 ("X axis value"), "X axis value"=0.0, "RobotDriveDevRef"=w277) -> ("error out"=w272:errorcluster, "Motor Values"=w274:dbl[], "RobotDriveDevRef"=w276:T16)  [unwired: 1 in, 5 out]
            }
          }
          "Motor Values" <- w220
          n105 = call "Autonomous Encoder Read.vi"("error in (no error)"=w205) -> ("error out"=w207:errorcluster, "Encoder Direction"=→"Encoder Direction 2":string, "Encoder Distance"=→"S2 Encoder":dbl)  [unwired: 8 in]
          n106 = call "Switch0 Pressed.vi"("error in (no error)"=w207) -> ("error out"=w206:errorcluster, "Switch Pressed"=w179:bool)  [unwired: 9 in]
          n107 = call-poly <vilib>:"NT Write Value.vi"("Numeric Array"=w220, "Name"="RobotDrive Motors") -> ()  [unwired: 9 in, 1 out]
          n108 = call <vilib>:"WPI_RobotDriveDelayAndUpdateSafety.vi"("error in (no error)"=w206, "Delay (s)"=5.0, "RobotDriveDevRef"=w222) -> ("RobotDriveDevRef 2"=w223:T16)  [unwired: 7 in, 1 out]
          n109 = Not(x=w179) -> (.not. x?=→"Move forward? S2":bool)
          n110 = case shown="False" w179 {
            tunnel: [w258 w265] -> w196
            tunnel: w223 -> [w259 w264]
            tunnel: [w257 w261] -> w188
            frame False {
              w255 = 45.0 ("desired angle")
              n111 = call "turning with gyro.vi"("desired angle"=w255, "RobotDriveDevRef"=w259) -> ("error out"=w257:errorcluster, "RobotDriveDevRef 2"=w258:T16)  [unwired: 8 in]
              n112 = call-poly <vilib>:"NT Write Value.vi"("Numeric"=w255, "Name"="Command Angle") -> ()  [unwired: 9 in, 1 out]
              "Step 1" <- TRUE
            }
            frame True {
              n113 = call-poly <vilib>:"WPI_RobotDriveArcadeDrive.vi"("Y axis value"=0.0 ("X axis value"), "X axis value"=0.0, "RobotDriveDevRef"=w264) -> ("error out"=w261:errorcluster, "RobotDriveDevRef"=w265:T16)  [unwired: 1 in, 6 out]
            }
          }
          n114 = call "read gyro.vi"("error in (no error)"=w188) -> ("Angle 2"=→"gyro step two":dbl)  [unwired: 9 in, 1 out]
          n115 = call "Switch0 Pressed.vi"("error in (no error)"=w188) -> ("Switch Pressed"=w178:bool)  [unwired: 9 in, 1 out]
          n116 = Not(x=w178) -> (.not. x?=→"Move forward? S 3":bool)
          n117 = case shown="False" FALSE {
            tunnel: w196 -> [w249 w254]
            tunnel: [w247 w251] -> w221
            tunnel: [w248 w250] -> w217
            frame False {
              n118 = call-poly <vilib>:"WPI_RobotDriveArcadeDrive.vi"("Y axis value"=-0.4 ("X axis value"), "X axis value"=0.0, "RobotDriveDevRef"=w249) -> ("Motor Values"=w247:dbl[], "RobotDriveDevRef"=w248:T16)  [unwired: 1 in, 6 out]
              "Step 2" <- TRUE
            }
            frame True {
              n119 = call-poly <vilib>:"WPI_RobotDriveArcadeDrive.vi"("Y axis value"=0.0 ("X axis value"), "X axis value"=0.0, "RobotDriveDevRef"=w254) -> ("Motor Values"=w251:dbl[], "RobotDriveDevRef"=w250:T16)  [unwired: 1 in, 6 out]
            }
          }
          n120 = flat-sequence {
            tunnel: w217 -> [w231]
            tunnel: [w231] -> w200
            tunnel: [w232] -> w199
            frame #0 {
              n121 = call "read gyro.vi"() -> ("Angle 2"=w232:dbl)  [unwired: 10 in, 1 out]
            }
          }
          n122 = case shown="False" FALSE {
            tunnel: [w238 w241] -> w197
            tunnel: w200 -> [w237 w240]
            tunnel: [w235 w239] -> w184
            frame False {
              w234 = 10.0 ("X axis value")
              n123 = call-poly <vilib>:"NT Write Value.vi"("Numeric"=w234, "Name"="Command Angle") -> ()  [unwired: 9 in, 1 out]
              n124 = call "turning with gyro.vi"("desired angle"=w234, "RobotDriveDevRef"=w237) -> ("error out"=w235:errorcluster, "RobotDriveDevRef 2"=w238:T16)  [unwired: 8 in]
              "Step 3" <- TRUE
            }
            frame True {
              n125 = call-poly <vilib>:"WPI_RobotDriveArcadeDrive.vi"("Y axis value"=0.0 ("X axis value"), "X axis value"=0.0, "RobotDriveDevRef"=w240) -> ("error out"=w239:errorcluster, "RobotDriveDevRef"=w241:T16)  [unwired: 1 in, 6 out]
            }
          }
          n126 = call "read gyro.vi"("error in (no error)"=w184) -> ("Angle 2"=→"gyro step  four":dbl)  [unwired: 9 in, 1 out]
          n127 = call-poly <vilib>:"NT Write Value.vi"("Numeric Array"=w221, "Name"=w216) -> ()  [unwired: 9 in, 1 out]
          n128 = flat-sequence {
            tunnel: w184 -> [_]
            tunnel: [w227] -> w176
            frame #0 {
              n129 = global read "Robot Global Data.vi" "Hook Center"() -> (→"Initial Hook Center 2":dbl)
              n130 = global read "Robot Global Data.vi" "Hook Found"() -> (w227:bool)
              "Initial Hook Found" <- w227
            }
          }
          n131 = call "search for hook.vi"("RobotDriveDevRef in"=w197, "Hook Found"=w176) -> ("error out"=w195:errorcluster, "Pixels to turn"=→"Pixels to turn":dbl, "RobotDriveDevRef out"=w194:T16, "Move forward? S 5"=→"Move forward? S 5":bool, "Hook found"=→"Hook found":bool, "Hook Found In False Case 2"=→"Hook Found In False Case 2":bool, "Degrees to turn"=→"Degrees to turn":dbl, "Hook Center"=→"Hook Center":dbl)  [unwired: 2 in]
          n132 = call "read distance.vi"("error in (no error)"=w195) -> ("Distance 2"=w192:dbl)  [unwired: 9 in, 1 out]
          "Distance to wall (in)" <- w192
          n133 = Subtract(x=w192, y=12.0) -> (x-y=w189:dbl)
          n134 = Less Than 0?(x=w189) -> (x < 0?=w191:bool)
          n135 = case shown="True" w191 {
            tunnel: [w229 1.0 ("f")] -> w190
            tunnel: w189 -> [w229 _]
            frame False {
            }
            frame True {
            }
          }
          n136 = call "drive forward.vi"("desired distance"=w190, "RobotDriveDevRef in"=w194) -> ("RobotDriveDevRef out"=w187:T16)  [unwired: 8 in, 1 out]
          n137 = call-poly <vilib>:"WPI_RobotDriveArcadeDrive.vi"("Y axis value"=0.0 ("X axis value"), "X axis value"=0.0, "RobotDriveDevRef"=w187) -> ("Motor Values"=w215:dbl[], "RobotDriveDevRef"=w185:T16)  [unwired: 1 in, 6 out]
          n138 = call <vilib>:"WPI_RobotDriveDelayAndUpdateSafety.vi"("Delay (s)"=1.0, "RobotDriveDevRef"=w185) -> ()  [unwired: 8 in, 2 out]
          n139 = call-poly <vilib>:"NT Write Value.vi"("Numeric Array"=w215, "Name"=w216) -> ()  [unwired: 9 in, 1 out]
          "gyro step  three" <- w199
          "Move forward? S4" <- TRUE ("Move forward? S4")
        }
      }
    }
  }
  n140 = disable-structure shown="Enabled" {
    frame Disabled {
      # "This tells you the autonomous selected\nfrom the dashboard"
      # "Every 20ms, report that we are running autonomous\ncode. Loop will abort the same time as the VI."
      # "Use time and/or sensors to control how the robot drives."
      # "This tells you the driver position\nand alliance color"
      n141 = while {
        stop <- FALSE stop-if-true
        n142 = Wait (ms)(milliseconds to wait=u32 20) -> ()  [unwired: 1 out]
        n143 = call <vilib>:"WPI_DriverStationReport Robot Code State.vi"("Autonomous"=TRUE) -> ()  [unwired: 10 in, 1 out]
      }
      n144 = call-poly <vilib>:"NT Read Value.vi"("Name"="Auto Selector") -> ("String"=w280:string)  [unwired: 9 in, 1 out]
      n145 = call <vilib>:"WPI_DriverStationGet Alliance Info.vi"() -> ("Position"=w279:T15)  [unwired: 11 out]
      n146 = case shown="Default" w280 {
        selector: w280 -> [_ _ w311]
        tunnel: w279 -> [_ _ _]
        frame "Alternative 1" {
          # "This sample code describes robot movements in an array. You can extend it to control other motors\non your robot. You can also use file I/O to move the data to a text file."
          n147 = call <vilib>:"WPI_RobotDriveRefNum Registry Get.vi"("refnum name"="Left and Right Motors") -> ("RobotDriveDevRef"=w282:T16)  [unwired: 1 in, 9 out]
          n148 = for {
            shift-right: [w290] -> _
            shift-left: w282 -> [w291]
            tunnel: "Array of robot movements 2" -> [w286] mode=indexing
            n149 = Unbundle By Name(w286) -> ("X Joystick Value"=w289:dbl, "Y Joystick Value"=w288:dbl, "Delay (sec)"=w287:dbl)  [unwired: 1 out]
            n150 = call-poly <vilib>:"WPI_RobotDriveArcadeDrive.vi"("Y axis value"=w288, "X axis value"=w289, "RobotDriveDevRef"=w291) -> ("Motor Values"=w284:dbl[], "RobotDriveDevRef"=w292:T16)  [unwired: 1 in, 6 out]
            n151 = call <vilib>:"WPI_RobotDriveDelayAndUpdateSafety.vi"("Delay (s)"=w287, "RobotDriveDevRef"=w292) -> ("RobotDriveDevRef 2"=w290:T16)  [unwired: 8 in, 1 out]
            n152 = call-poly <vilib>:"NT Write Value.vi"("Numeric Array"=w284, "Name"="RobotDrive Motors") -> ()  [unwired: 9 in, 1 out]
            "Current Movement, for debugging 2" <- w286
          }
        }
        frame "Alternative 2" {
          w294 = "RobotDrive Motors" ("Name")
          # "This is some simple sample code to drive your robot curving one direction and then the other."
          # "stand still"
          # "other way for 0.5 second"
          # "turn for 1 second"
          n153 = call <vilib>:"WPI_RobotDriveRefNum Registry Get.vi"("refnum name"="Left and Right Motors") -> ("RobotDriveDevRef"=w310:T16)  [unwired: 1 in, 9 out]
          n154 = call-poly <vilib>:"WPI_RobotDriveArcadeDrive.vi"("Y axis value"=0.5 ("X axis value"), "X axis value"=-0.25, "RobotDriveDevRef"=w310) -> ("Motor Values"=w293:dbl[], "RobotDriveDevRef"=w303:T16)  [unwired: 1 in, 6 out]
          n155 = call <vilib>:"WPI_RobotDriveDelayAndUpdateSafety.vi"("Delay (s)"=1.0, "RobotDriveDevRef"=w303) -> ("RobotDriveDevRef 2"=w304:T16)  [unwired: 8 in, 1 out]
          n156 = call-poly <vilib>:"WPI_RobotDriveArcadeDrive.vi"("Y axis value"=-0.25 ("X axis value"), "X axis value"=0.5, "RobotDriveDevRef"=w304) -> ("Motor Values"=w295:dbl[], "RobotDriveDevRef"=w305:T16)  [unwired: 1 in, 6 out]
          n157 = call <vilib>:"WPI_RobotDriveDelayAndUpdateSafety.vi"("Delay (s)"=0.5, "RobotDriveDevRef"=w305) -> ("RobotDriveDevRef 2"=w306:T16)  [unwired: 8 in, 1 out]
          n158 = call-poly <vilib>:"NT Write Value.vi"("Numeric Array"=w293, "Name"=w294) -> ()  [unwired: 9 in, 1 out]
          n159 = call-poly <vilib>:"NT Write Value.vi"("Numeric Array"=w295, "Name"=w294) -> ()  [unwired: 9 in, 1 out]
          n160 = call-poly <vilib>:"WPI_RobotDriveArcadeDrive.vi"("Y axis value"=0.0 ("X axis value"), "X axis value"=0.0, "RobotDriveDevRef"=w306) -> ("Motor Values"=w296:dbl[])  [unwired: 1 in, 7 out]
          n161 = call-poly <vilib>:"NT Write Value.vi"("Numeric Array"=w296, "Name"=w294) -> ()  [unwired: 9 in, 1 out]
        }
        frame Default {
          n162 = case shown="\"True\"" w311 {
            frame "False", Default {
            }
            frame "True" {
              w324 = FPGA_DIOChannel."DIO 1"  # B Channel
              w323 = FPGA_DIOChannel."DIO 0"  # A Channel
              w337 = FPGA_DIOChannel."DIO 1"  # B Channel
              w336 = FPGA_DIOChannel."DIO 0"  # A Channel
              w348 = FPGA_DIOChannel."DIO 1"  # B Channel
              w347 = FPGA_DIOChannel."DIO 0"  # A Channel
              w360 = FPGA_DIOChannel."DIO 1"  # B Channel
              w359 = FPGA_DIOChannel."DIO 0"  # A Channel
              w372 = FPGA_DIOChannel."DIO 1"  # B Channel
              w371 = FPGA_DIOChannel."DIO 0"  # A Channel
              w384 = FPGA_DIOChannel."DIO 1"  # B Channel
              w383 = FPGA_DIOChannel."DIO 0"  # A Channel
              w395 = FPGA_DIOChannel."DIO 1"  # B Channel
              w394 = FPGA_DIOChannel."DIO 0"  # A Channel
              (unwired) 0.0 ("Distance")
              # "in inches"
              # "in inches"
              # "in inches"
              # "in inches"
              # "in inches"
              # "in inches"
              # "in inches"
              n163 = call <vilib>:"WPI_DigitalInputOpen.vi"("DIO Channel"=w394) -> ("DigitalInputDevRef"=w391:T4)  [unwired: 1 in, 9 out]
              n164 = call <vilib>:"WPI_DigitalInputOpen.vi"("DIO Channel"=w395) -> ("DigitalInputDevRef"=w392:T4)  [unwired: 1 in, 9 out]
              n165 = call-poly <vilib>:"WPI_CounterToDigitalSource.vi"("DigitalInputDevRef"=w391) -> ("Digital Source"=w312:T5)  [unwired: 6 out]
              n166 = call-poly <vilib>:"WPI_CounterToDigitalSource.vi"("DigitalInputDevRef"=w392) -> ("Digital Source"=w393:T5)  [unwired: 6 out]
              n167 = call <vilib>:"WPI_EncoderOpen.vi"("DistancePerCount"=18.84955592153876, "BSource"=w393, "ASource"=w312) -> ("error out"=w388:errorcluster, "EncoderDevRef"=w389:T9)  [unwired: 5 in, 2 out]
              n168 = call <vilib>:"WPI_EncoderGet.vi"("error in (no error)"=w388, "EncoderDevRef"=w389) -> ("Distance"=w387:dbl)  [unwired: 4 in, 5 out]
              n169 = call <vilib>:"WPI_RobotDriveRefNum Registry Get.vi"("refnum name"="Left Right Motors") -> ("RobotDriveDevRef"=w414:T16)  [unwired: 9 in, 1 out]
              n170 = Equal?(x=w387, y=100.0) -> (x = y?=w385:bool)
              n171 = case shown="True" w385 {
                tunnel: w414 -> [w444 w448]
                tunnel: [w444 w445] -> w413
                frame False {
                }
                frame True {
                  n172 = call-poly <vilib>:"WPI_RobotDriveArcadeDrive.vi"("Y axis value"=0.05, "X axis value"=0.0, "RobotDriveDevRef"=w448) -> ("RobotDriveDevRef"=w445:T16)  [unwired: 6 in, 2 out]
                }
              }
              n173 = call <vilib>:"WPI_DigitalInputOpen.vi"("DIO Channel"=w383) -> ("DigitalInputDevRef"=w380:T4)  [unwired: 1 in, 9 out]
              n174 = call <vilib>:"WPI_DigitalInputOpen.vi"("DIO Channel"=w384) -> ("DigitalInputDevRef"=w381:T4)  [unwired: 1 in, 9 out]
              n175 = call-poly <vilib>:"WPI_CounterToDigitalSource.vi"("DigitalInputDevRef"=w380) -> ("Digital Source"=w379:T5)  [unwired: 6 out]
              n176 = call-poly <vilib>:"WPI_CounterToDigitalSource.vi"("DigitalInputDevRef"=w381) -> ("Digital Source"=w382:T5)  [unwired: 6 out]
              n177 = call <vilib>:"WPI_EncoderOpen.vi"("DistancePerCount"=18.84955592153876, "BSource"=w382, "ASource"=w379) -> ("error out"=w376:errorcluster, "EncoderDevRef"=w377:T9)  [unwired: 5 in, 2 out]
              n178 = call <vilib>:"WPI_EncoderGet.vi"("error in (no error)"=w376, "EncoderDevRef"=w377) -> ("Distance"=w375:dbl)  [unwired: 4 in, 5 out]
              n179 = call <vilib>:"WPI_RobotDriveDelayAndUpdateSafety.vi"("Delay (s)"=0.07, "RobotDriveDevRef"=w413) -> ("RobotDriveDevRef 2"=w409:T16)  [unwired: 8 in, 1 out]
              n180 = Equal?(x=w375, y=100.0) -> (x = y?=w373:bool)
              n181 = case shown="True" w373 {
                tunnel: w409 -> [w439 w443]
                tunnel: [w439 w440] -> w411
                frame False {
                }
                frame True {
                  n182 = call-poly <vilib>:"WPI_RobotDriveArcadeDrive.vi"("Y axis value"=0.15, "X axis value"=0.0, "RobotDriveDevRef"=w443) -> ("RobotDriveDevRef"=w440:T16)  [unwired: 6 in, 2 out]
                }
              }
              n183 = call <vilib>:"WPI_DigitalInputOpen.vi"("DIO Channel"=w371) -> ("DigitalInputDevRef"=w368:T4)  [unwired: 1 in, 9 out]
              n184 = call <vilib>:"WPI_DigitalInputOpen.vi"("DIO Channel"=w372) -> ("DigitalInputDevRef"=w369:T4)  [unwired: 1 in, 9 out]
              n185 = call-poly <vilib>:"WPI_CounterToDigitalSource.vi"("DigitalInputDevRef"=w368) -> ("Digital Source"=w367:T5)  [unwired: 6 out]
              n186 = call-poly <vilib>:"WPI_CounterToDigitalSource.vi"("DigitalInputDevRef"=w369) -> ("Digital Source"=w370:T5)  [unwired: 6 out]
              n187 = call <vilib>:"WPI_EncoderOpen.vi"("DistancePerCount"=18.84955592153876, "BSource"=w370, "ASource"=w367) -> ("error out"=w364:errorcluster, "EncoderDevRef"=w365:T9)  [unwired: 5 in, 2 out]
              n188 = call <vilib>:"WPI_EncoderGet.vi"("error in (no error)"=w364, "EncoderDevRef"=w365) -> ("Distance"=w363:dbl)  [unwired: 4 in, 5 out]
              n189 = call <vilib>:"WPI_RobotDriveDelayAndUpdateSafety.vi"("Delay (s)"=0.1, "RobotDriveDevRef"=w411) -> ("RobotDriveDevRef 2"=w406:T16)  [unwired: 8 in, 1 out]
              n190 = Equal?(x=w363, y=100.0) -> (x = y?=w361:bool)
              n191 = case shown="True" w361 {
                tunnel: w406 -> [w434 w438]
                tunnel: [w434 w435] -> w408
                frame False {
                }
                frame True {
                  n192 = call-poly <vilib>:"WPI_RobotDriveArcadeDrive.vi"("Y axis value"=0.3, "X axis value"=0.0, "RobotDriveDevRef"=w438) -> ("RobotDriveDevRef"=w435:T16)  [unwired: 6 in, 2 out]
                }
              }
              n193 = call <vilib>:"WPI_DigitalInputOpen.vi"("DIO Channel"=w359) -> ("DigitalInputDevRef"=w356:T4)  [unwired: 1 in, 9 out]
              n194 = call <vilib>:"WPI_DigitalInputOpen.vi"("DIO Channel"=w360) -> ("DigitalInputDevRef"=w357:T4)  [unwired: 1 in, 9 out]
              n195 = call-poly <vilib>:"WPI_CounterToDigitalSource.vi"("DigitalInputDevRef"=w356) -> ("Digital Source"=w355:T5)  [unwired: 6 out]
              n196 = call-poly <vilib>:"WPI_CounterToDigitalSource.vi"("DigitalInputDevRef"=w357) -> ("Digital Source"=w358:T5)  [unwired: 6 out]
              n197 = call <vilib>:"WPI_EncoderOpen.vi"("DistancePerCount"=18.84955592153876, "BSource"=w358, "ASource"=w355) -> ("error out"=w352:errorcluster, "EncoderDevRef"=w353:T9)  [unwired: 5 in, 2 out]
              n198 = call <vilib>:"WPI_EncoderGet.vi"("error in (no error)"=w352, "EncoderDevRef"=w353) -> ("Distance"=w351:dbl)  [unwired: 4 in, 5 out]
              n199 = call <vilib>:"WPI_RobotDriveDelayAndUpdateSafety.vi"("Delay (s)"=0.1, "RobotDriveDevRef"=w408) -> ("RobotDriveDevRef 2"=w404:T16)  [unwired: 8 in, 1 out]
              n200 = Equal?(x=w351, y=100.0) -> (x = y?=w349:bool)
              n201 = case shown="True" w349 {
                tunnel: w404 -> [w429 w433]
                tunnel: [w429 w430] -> w405
                frame False {
                }
                frame True {
                  n202 = call-poly <vilib>:"WPI_RobotDriveArcadeDrive.vi"("Y axis value"=0.5, "X axis value"=0.0, "RobotDriveDevRef"=w433) -> ("RobotDriveDevRef"=w430:T16)  [unwired: 6 in, 2 out]
                }
              }
              n203 = call <vilib>:"WPI_DigitalInputOpen.vi"("DIO Channel"=w347) -> ("DigitalInputDevRef"=w344:T4)  [unwired: 1 in, 9 out]
              n204 = call <vilib>:"WPI_DigitalInputOpen.vi"("DIO Channel"=w348) -> ("DigitalInputDevRef"=w345:T4)  [unwired: 1 in, 9 out]
              n205 = call-poly <vilib>:"WPI_CounterToDigitalSource.vi"("DigitalInputDevRef"=w344) -> ("Digital Source"=w343:T5)  [unwired: 6 out]
              n206 = call-poly <vilib>:"WPI_CounterToDigitalSource.vi"("DigitalInputDevRef"=w345) -> ("Digital Source"=w346:T5)  [unwired: 6 out]
              n207 = call <vilib>:"WPI_EncoderOpen.vi"("DistancePerCount"=18.84955592153876, "BSource"=w346, "ASource"=w343) -> ("error out"=w340:errorcluster, "EncoderDevRef"=w341:T9)  [unwired: 5 in, 2 out]
              n208 = call <vilib>:"WPI_EncoderGet.vi"("error in (no error)"=w340, "EncoderDevRef"=w341) -> ("Distance"=w339:dbl)  [unwired: 4 in, 5 out]
              n209 = call <vilib>:"WPI_RobotDriveDelayAndUpdateSafety.vi"("Delay (s)"=0.1, "RobotDriveDevRef"=w405) -> ("RobotDriveDevRef 2"=w400:T16)  [unwired: 8 in, 1 out]
              n210 = Equal?(x=w339, y=100.0) -> (x = y?=w326:bool)
              n211 = case shown="True" w326 {
                tunnel: w400 -> [w424 w428]
                tunnel: [w424 w425] -> w401
                frame False {
                }
                frame True {
                  n212 = call-poly <vilib>:"WPI_RobotDriveArcadeDrive.vi"("Y axis value"=0.7, "X axis value"=0.0, "RobotDriveDevRef"=w428) -> ("RobotDriveDevRef"=w425:T16)  [unwired: 6 in, 2 out]
                }
              }
              n213 = call <vilib>:"WPI_DigitalInputOpen.vi"("DIO Channel"=w336) -> ("DigitalInputDevRef"=w333:T4)  [unwired: 1 in, 9 out]
              n214 = call <vilib>:"WPI_DigitalInputOpen.vi"("DIO Channel"=w337) -> ("DigitalInputDevRef"=w334:T4)  [unwired: 1 in, 9 out]
              n215 = call-poly <vilib>:"WPI_CounterToDigitalSource.vi"("DigitalInputDevRef"=w333) -> ("Digital Source"=w332:T5)  [unwired: 6 out]
              n216 = call-poly <vilib>:"WPI_CounterToDigitalSource.vi"("DigitalInputDevRef"=w334) -> ("Digital Source"=w335:T5)  [unwired: 6 out]
              n217 = call <vilib>:"WPI_EncoderOpen.vi"("DistancePerCount"=18.84955592153876, "BSource"=w335, "ASource"=w332) -> ("error out"=w329:errorcluster, "EncoderDevRef"=w330:T9)  [unwired: 5 in, 2 out]
              n218 = call <vilib>:"WPI_EncoderGet.vi"("error in (no error)"=w329, "EncoderDevRef"=w330) -> ("Distance"=w328:dbl)  [unwired: 4 in, 5 out]
              n219 = call <vilib>:"WPI_RobotDriveDelayAndUpdateSafety.vi"("Delay (s)"=0.1, "RobotDriveDevRef"=w401) -> ("RobotDriveDevRef 2"=w397:T16)  [unwired: 8 in, 1 out]
              n220 = Equal?(x=w328, y=100.0) -> (x = y?=w325:bool)
              n221 = case shown="True" w325 {
                tunnel: w397 -> [w419 w423]
                tunnel: [w419 w420] -> w398
                frame False {
                }
                frame True {
                  n222 = call-poly <vilib>:"WPI_RobotDriveArcadeDrive.vi"("Y axis value"=0.9, "X axis value"=0.0, "RobotDriveDevRef"=w423) -> ("RobotDriveDevRef"=w420:T16)  [unwired: 6 in, 2 out]
                }
              }
              n223 = call <vilib>:"WPI_DigitalInputOpen.vi"("DIO Channel"=w323) -> ("DigitalInputDevRef"=w320:T4)  [unwired: 1 in, 9 out]
              n224 = call <vilib>:"WPI_DigitalInputOpen.vi"("DIO Channel"=w324) -> ("DigitalInputDevRef"=w321:T4)  [unwired: 1 in, 9 out]
              n225 = call-poly <vilib>:"WPI_CounterToDigitalSource.vi"("DigitalInputDevRef"=w320) -> ("Digital Source"=w319:T5)  [unwired: 6 out]
              n226 = call-poly <vilib>:"WPI_CounterToDigitalSource.vi"("DigitalInputDevRef"=w321) -> ("Digital Source"=w322:T5)  [unwired: 6 out]
              n227 = call <vilib>:"WPI_EncoderOpen.vi"("DistancePerCount"=18.84955592153876, "BSource"=w322, "ASource"=w319) -> ("error out"=w316:errorcluster, "EncoderDevRef"=w317:T9)  [unwired: 5 in, 2 out]
              n228 = call <vilib>:"WPI_EncoderGet.vi"("error in (no error)"=w316, "EncoderDevRef"=w317) -> ("Distance"=w315:dbl)  [unwired: 4 in, 5 out]
              n229 = call <vilib>:"WPI_RobotDriveDelayAndUpdateSafety.vi"("Delay (s)"=0.1, "RobotDriveDevRef"=w398) -> ("RobotDriveDevRef 2"=w396:T16)  [unwired: 8 in, 1 out]
              n230 = Equal?(x=w315, y=100.0) -> (x = y?=w313:bool)
              n231 = case shown="True" w313 {
                tunnel: w396 -> [_ w418]
                frame False {
                }
                frame True {
                  n232 = call-poly <vilib>:"WPI_RobotDriveArcadeDrive.vi"("Y axis value"=0.5, "X axis value"=0.0, "RobotDriveDevRef"=w418) -> ()  [unwired: 6 in, 3 out]
                }
              }
            }
          }
        }
      }
    }
    frame Enabled {
    }
  }
  n233 = Index Array(array=w3, index #1=2 ("index")) -> ()  [unwired: 1 in, 2 out]
  n234 = call-poly <vilib>:"NT Write Value.vi"("Numeric Array"=w3, "Name"="Joystick 0/Axes") -> ()  [unwired: 9 in, 1 out]
